vi "Generate Actual Voltage.vi"(0 "Ideal Voltage":dbl[](array[numeric]), 5 "Error Percentage":dbl, 11 "Error In":errorcluster) -> (4 "Actual Voltage":dbl[](array[numeric]), 15 "Error Out":errorcluster)   [LabVIEW 2023]
doc: "The VI introduces the given percentage of error into the ideal voltage and generate actual voltage."
uses:
  <vilib>/numeric/Random Number (Range) DBL.vi
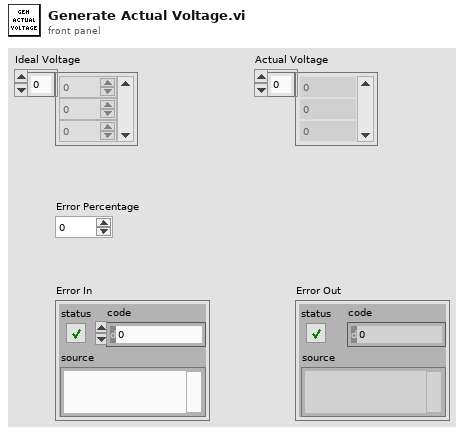
[diagram p1: front panel]
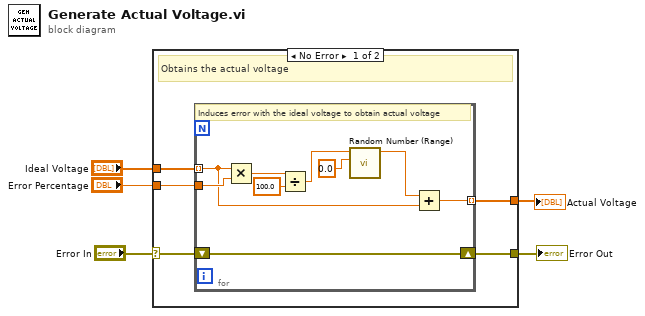
[diagram p0: block diagram]
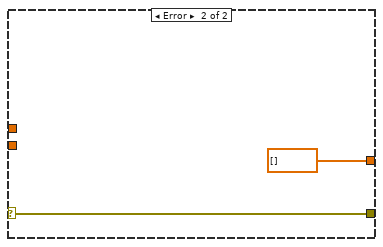
[diagram p2: hidden frame]
diagram:
  n1 = case shown="No Error" "Error In" {
    selector: "Error In" -> [w10 w20]
    tunnel: [w9 w20] -> w4
    tunnel: [w8 dbl[] []] -> w3
    tunnel: "Error Percentage" -> [w7 _]
    tunnel: "Ideal Voltage" -> [w6 _]
    frame No Error {
      # "Obtains the actual voltage"
      n2 = for {
        tunnel: w6 -> [w12] mode=indexing
        tunnel: w7 -> [w19]
        tunnel: [w13] -> w8 mode=indexing
        shift-right: [w14] -> w9
        shift-left: w10 -> [w14]
        # "Induces error with the ideal voltage to obtain actual voltage"
        n3 = Multiply(x=w12, y=w19) -> (x*y=w18:dbl)
        n4 = Divide(x=w18, y=100.0) -> (x/y=w15:dbl)
        n5 = call-poly <vilib>:"Random Number (Range).vi"("lower bound (0)"=0.0, "upper bound (100)"=w15) -> ("number"=w11:dbl)  [unwired: 9 in]
        n6 = Add(x=w11, y=w12) -> (x+y=w13:dbl)
      }
    }
    frame Error {
    }
  }
  "Error Out" <- w4
  "Actual Voltage" <- w3
